vi "write read Lens Driver.vi"(0 "VISA resource name":refnum<visa-resource-name>, 5 "command":string, 7 "Calibration":T1 {"Max Current A" format="%#_g mA"; "Max Current B" format="%#_g mA"; "UCL A" format="%#_g mA"; "LCL A" format="%#_g mA"; "UCL B" format="%#_g mA"; "LCL B" format="%#_g mA"}, 11 "error in (no error)":errorcluster) -> (2 "M":i32, 4 "VISA resource name out":refnum<visa-resource-name>, 6 "Calibration 2":T1 {"Max Current A" format="%#_g mA"; "Max Current B" format="%#_g mA"; "UCL A" format="%#_g mA"; "LCL A" format="%#_g mA"; "UCL B" format="%#_g mA"; "LCL B" format="%#_g mA"}, 8 "OK":bool, 10 "Data":string, 12 "TA":u16, 13 "TB":u16, 15 "error out":errorcluster)   [LabVIEW 2024]
doc: "Basic VI to write a command to the Lens Driver and read back the answer.\nOptotune AG, 2014"
uses:
  Calibration.ctl
panel:
  out "i":i32
  out "C value":i16
  out "Number of Bytes at Serial Port":u32
  out "elapsed time (ms)":u32
  out "Response":string
  out "write":string
  out "CRC16":string
  out "read buffer":string
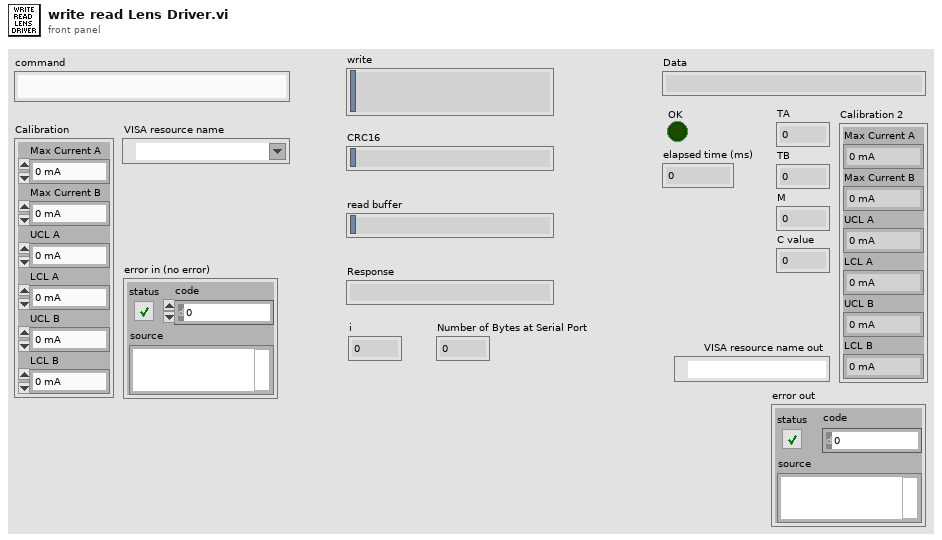
[diagram p1: front panel]
types:
  T1 = typedef "Calibration.ctl" = cluster{"Max Current A":dbl, "Max Current B":dbl, "UCL A":dbl, "UCL B":dbl, "LCL A":dbl, "LCL B":dbl}
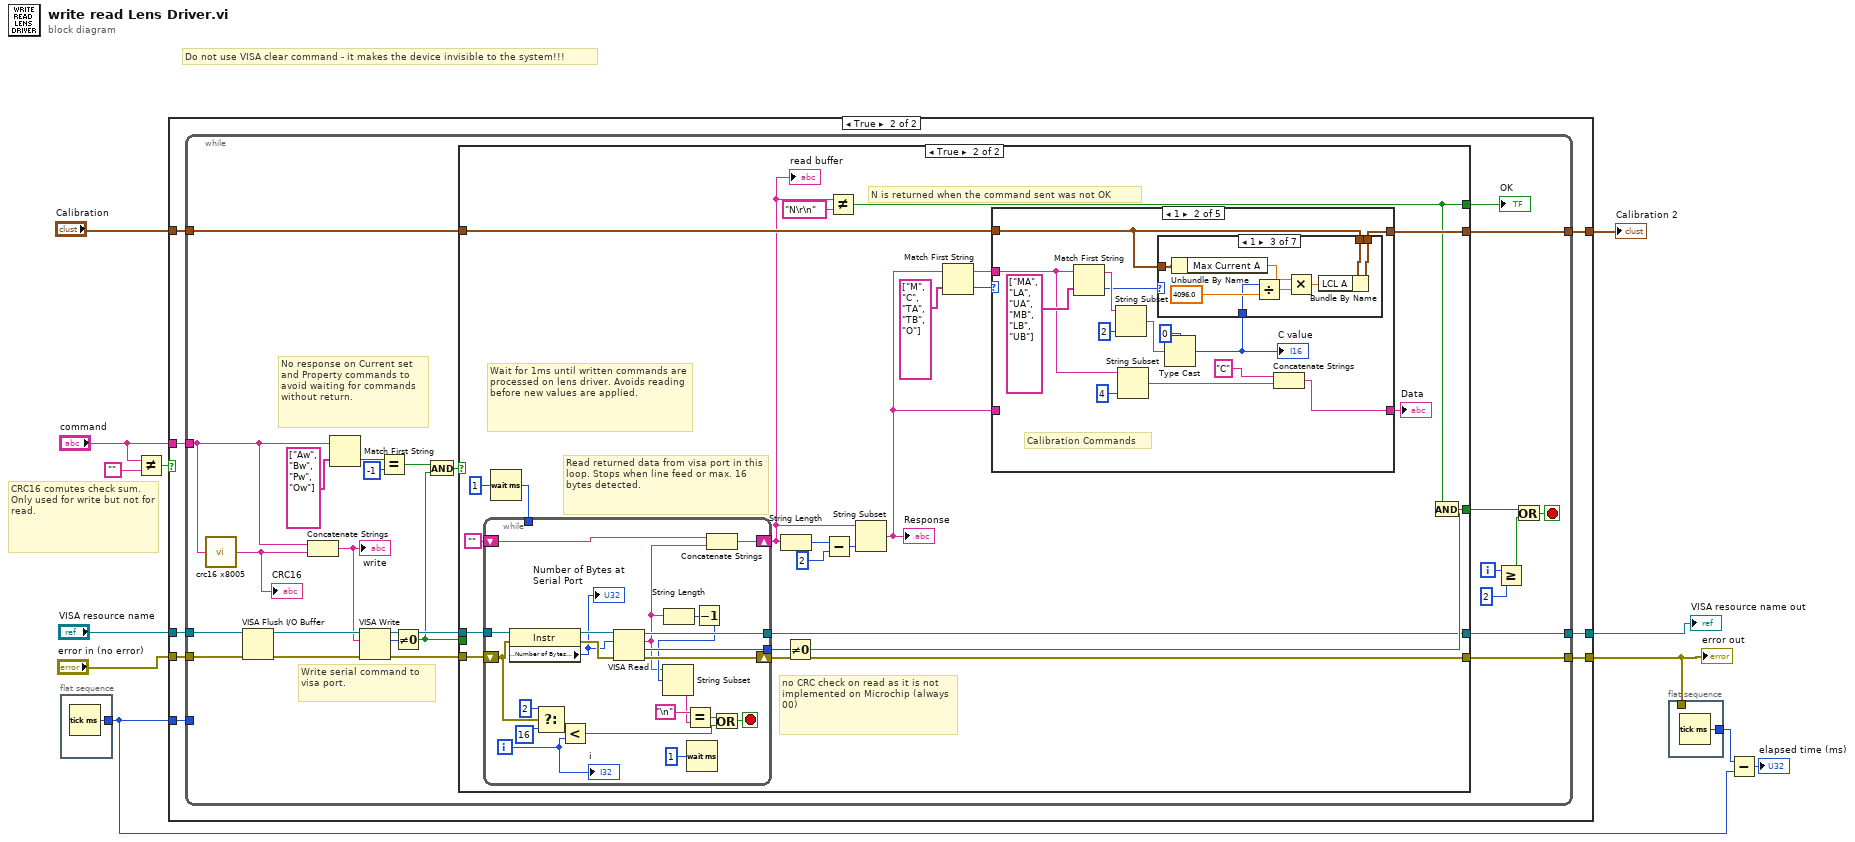
[diagram p0: block diagram]
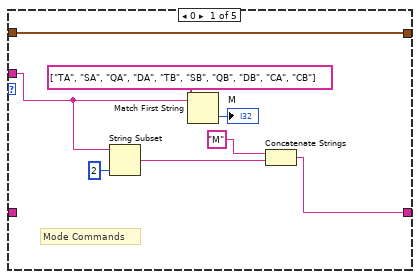
[diagram p4: hidden frame]
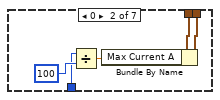
[diagram p6: hidden frame]
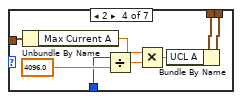
[diagram p7: hidden frame]
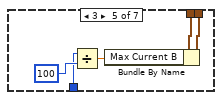
[diagram p8: hidden frame]
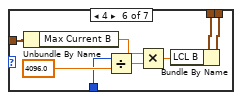
[diagram p9: hidden frame]
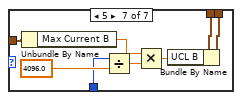
[diagram p10: hidden frame]
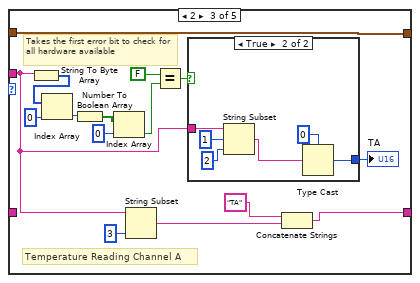
[diagram p11: hidden frame]
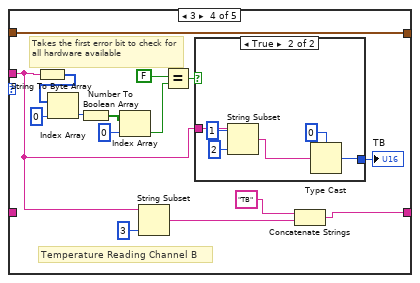
[diagram p13: hidden frame]
diagram:
  # "CRC16 comutes check sum. Only used for write but not for read."
  # "Do not use VISA clear command - it makes the device invisible to the system!!!"
  n1 = flat-sequence {
    tunnel: [w13] -> _
    tunnel: [w13] -> w10
    frame #0 {
      n2 = Tick Count (ms)() -> (millisecond timer value=w13:u32)
    }
  }
  n3 = Not Equal?(x="command", y="") -> (x != y?=w6:bool)
  n4 = case shown="True" w6 {
    tunnel: w10 -> [_ w24]
    tunnel: [w14 w23] -> w9
    tunnel: [w15 w22] -> w8
    tunnel: "Calibration" -> [w16 w21]
    tunnel: [w16 w20] -> w7
    tunnel: "command" -> [_ w19]
    tunnel: "VISA resource name" -> [w15 w18]
    tunnel: "error in (no error)" -> [w14 w17]
    frame False {
    }
    frame True {
      n5 = while {
        tunnel: w24 -> [_]
        tunnel: [w39] -> w23
        tunnel: [w35] -> w22
        tunnel: w21 -> [w30]
        tunnel: [w29] -> w20
        tunnel: w19 -> [w27]
        tunnel: w18 -> [w26]
        tunnel: w17 -> [w25]
        i -> [w33]
        stop <- w34 stop-if-true
        # "Write serial command to visa port."
        # "No response on Current set and Property commands to avoid waiting for commands without return."
        n6 = call "crc16 x8005.vi"("message"=w27) -> ("CRC16"=w45:string)  [unwired: 4 in]
        "CRC16" <- w45
        n7 = VISA Flush I/O Buffer(VISA resource name=w26, error in (no error)=w25) -> (VISA resource name out=w47:refnum<visa-resource-name>, error out=w46:errorcluster)  [unwired: 1 in]
        n8 = Concatenate Strings(w27, w45) -> (w44:string)
        "write" <- w44
        n9 = Match First String(2:string[] ["Aw", "Bw", "Pw", "Ow"] ("string array"), 3:w27) -> (0:w42:i32)  [unwired: 1 out]
        n10 = VISA Write(VISA resource name=w47, write buffer=w44, error in (no error)=w46) -> (VISA resource name out=w50:refnum<visa-resource-name>, return count=w38:u32, error out=w48:errorcluster)
        n11 = Equal?(x=w42, y=-1) -> (x = y?=w40:bool)
        n12 = Not Equal To 0?(x=w38) -> (x != 0?=w36:bool)
        n13 = And(x=w40, y=w36) -> (x .and. y?=w37:bool)
        n14 = case shown="True" w37 {
          tunnel: w50 -> [w53 w75]
          tunnel: [w51 w73] -> w49
          tunnel: w48 -> [w54 w72]
          tunnel: [w54 w69] -> w39
          tunnel: w36 -> [w51 _]
          tunnel: [w53 w63] -> w35
          tunnel: w30 -> [w52 w61]
          tunnel: [w52 w60] -> w29
          tunnel: [w51 w59] -> w28
          frame False {
          }
          frame True {
            # "Wait for 1ms until written commands are processed on lens driver. Avoids reading before new values are applied."
            # "Read returned data from visa port in this loop. Stops when line feed or max. 16 bytes detected."
            # "N is returned when the command sent was not OK"
            # "no CRC check on read as it is not implemented on Microchip (always 00)"
            n15 = Wait (ms)(milliseconds to wait=u32 1) -> (millisecond timer value=w55:u32)
            n16 = while {
              tunnel: w75 -> [w203]
              tunnel: [w208] -> w63
              shift-right: [w205] -> w57
              shift-left: "" -> [w204]
              tunnel: [w197] -> w65
              shift-right: [w209] -> w69
              shift-left: w72 -> [w193]
              tunnel: w55 -> [_]
              i -> [w199]
              stop <- w201 stop-if-true
              n17 = property class="Instr"(reference=w203, error in=w193) -> (reference out=w198:refnum<visa-resource-name>, error out=w196:errorcluster, "Serial Settings:Number of Bytes at Serial Port"=w192:u32)
              "Number of Bytes at Serial Port" <- w192
              n18 = Select(t=2, s=w193, f=16 ("x")) -> (s? t:f=w195:i32)
              n19 = Less?(x=w195, y=w199) -> (x < y?=w200:bool)
              n20 = VISA Read(VISA resource name=w198, byte count=w192, error in (no error)=w196) -> (VISA resource name out=w208:refnum<visa-resource-name>, read buffer=w188:string, return count=w197:u32, error out=w209:errorcluster)
              n21 = String Length(string=w188) -> (length=w190:i32)
              n22 = Wait (ms)(milliseconds to wait=u32 1) -> ()  [unwired: 1 out]
              n23 = Decrement(x=w190) -> (x-1=w189:i32)
              n24 = String Subset(string=w188, offset (0)=w189) -> (substring=w191:string)  [unwired: 1 in]
              n25 = Equal?(x="\n", y=w191) -> (x = y?=w206:bool)
              n26 = Concatenate Strings(w204, w188) -> (w205:string)
              n27 = Or(x=w206, y=w200) -> (x .or. y?=w201:bool)
              "i" <- w199
            }
            "read buffer" <- w57
            n28 = String Length(string=w57) -> (length=w76:i32)
            n29 = Not Equal To 0?(x=w65) -> (x != 0?=w64:bool)
            n30 = Subtract(x=w76, y=2) -> (x-y=w77:i32)
            n31 = Not Equal?(x=w57, y="N\r\n") -> (x != y?=w59:bool)
            n32 = String Subset(string=w57, length (rest)=w77) -> (substring=w58:string)  [unwired: 1 in]
            "Response" <- w58
            n33 = Match First String(2:string[] ["M", "C", "TA", "TB", "O"] ("string array"), 3:w58) -> (0:w67:i32, 1:w66:string)
            n34 = case shown="1" w67 {
              tunnel: w66 -> [w83 w93 w144 w164 _]
              tunnel: [w79 w92 w152 w173 w185] -> w62
              tunnel: [w78 w91 w151 w172 w186] -> w60
              tunnel: w61 -> [w78 w86 w151 w172 w186]
              tunnel: w58 -> [_ _ _ _ w185]
              frame 0 {
                # "Mode Commands"
                n35 = String Subset(string=w83, length (rest)=2 ("length (rest)")) -> (substring=w80:string)  [unwired: 1 in]
                n36 = Match First String(2:string[] ["TA", "SA", "QA", "DA", "TB", "SB", "QB", "DB", "CA", "CB"] ("string array"), 3:w83) -> (0:→"M":i32)  [unwired: 1 out]
                n37 = Concatenate Strings("M", w80) -> (w79:string)
              }
              frame 1 {
                # "Calibration Commands"
                n38 = Match First String(2:string[] ["MA", "LA", "UA", "MB", "LB", "UB"] ("string array"), 3:w93) -> (0:w90:i32, 1:w97:string)
                n39 = String Subset(string=w97, length (rest)=2 ("length (rest)")) -> (substring=w88:string)  [unwired: 1 in]
                n40 = String Subset(string=w93, length (rest)=4 ("length (rest)")) -> (substring=w94:string)  [unwired: 1 in]
                n41 = Type Cast(type=i16 0 ("length (rest)"), x=w88) -> (*(type *) &x=w87:i16)
                "C value" <- w87
                n42 = case shown="1" w90 {
                  tunnel: w86 -> [w100 w105 w113 w121 w126 w134 w142]
                  tunnel: [w100 w104 w112 w120 w125 w133 w141] -> w91
                  tunnel: w87 -> [_ w102 w106 w114 w122 w127 w135]
                  tunnel: w86 -> [_ _ w111 w115 _ w128 w136]
                  frame -1, Default {
                  }
                  frame 0 {
                    n43 = Divide(x=w102, y=u16 100) -> (x/y=w101:dbl)
                    n44 = Bundle By Name(cluster=w105, "Max Current A"=w101) -> (w104:T1)
                  }
                  frame 1 {
                    n45 = Unbundle By Name(w111) -> ("Max Current A"=w109:dbl)
                    n46 = Divide(x=w106, y=4096.0) -> (x/y=w107:dbl)
                    n47 = Multiply(x=w109, y=w107) -> (x*y=w108:dbl)
                    n48 = Bundle By Name(cluster=w113, "LCL A"=w108) -> (w112:T1)
                  }
                  frame 2 {
                    n49 = Unbundle By Name(w115) -> ("Max Current A"=w118:dbl)
                    n50 = Divide(x=w114, y=4096.0) -> (x/y=w117:dbl)
                    n51 = Multiply(x=w118, y=w117) -> (x*y=w116:dbl)
                    n52 = Bundle By Name(cluster=w121, "UCL A"=w116) -> (w120:T1)
                  }
                  frame 3 {
                    n53 = Divide(x=w122, y=u16 100) -> (x/y=w124:dbl)
                    n54 = Bundle By Name(cluster=w126, "Max Current B"=w124) -> (w125:T1)
                  }
                  frame 4 {
                    n55 = Unbundle By Name(w128) -> ("Max Current B"=w131:dbl)
                    n56 = Divide(x=w127, y=4096.0) -> (x/y=w130:dbl)
                    n57 = Multiply(x=w131, y=w130) -> (x*y=w129:dbl)
                    n58 = Bundle By Name(cluster=w134, "LCL B"=w129) -> (w133:T1)
                  }
                  frame 5 {
                    n59 = Unbundle By Name(w136) -> ("Max Current B"=w139:dbl)
                    n60 = Divide(x=w135, y=4096.0) -> (x/y=w140:dbl)
                    n61 = Multiply(x=w139, y=w140) -> (x*y=w137:dbl)
                    n62 = Bundle By Name(cluster=w142, "UCL B"=w137) -> (w141:T1)
                  }
                }
                n63 = Concatenate Strings("C", w94) -> (w92:string)
              }
              frame 2 {
                # "Takes the first error bit to check for all hardware available"
                # "Temperature Reading Channel A"
                n64 = String To Byte Array(string=w144) -> (unsigned byte array=w149:u8[])
                n65 = Index Array(array=w149, index=0) -> (element=w148:u8)
                n66 = Number To Boolean Array(number=w148) -> (Boolean array=w146:bool[])
                n67 = Index Array(array=w146, index=0) -> (element=w143:bool)
                n68 = String Subset(string=w144, length (rest)=3 ("length (rest)")) -> (substring=w153:string)  [unwired: 1 in]
                n69 = Equal?(x=FALSE, y=w143) -> (x = y?=w157:bool)
                n70 = case shown="True" w157 {
                  tunnel: w144 -> [_ w162]
                  tunnel: [_ w159] -> w156
                  frame False {
                  }
                  frame True {
                    n71 = String Subset(string=w162, offset (0)=1, length (rest)=2 ("length (rest)")) -> (substring=w158:string)
                    n72 = Type Cast(type=u16 0 ("length (rest)"), x=w158) -> (*(type *) &x=w159:u16)
                  }
                }
                "TA" <- w156
                n73 = Concatenate Strings("TA", w153) -> (w152:string)
              }
              frame 3 {
                # "Takes the first error bit to check for all hardware available"
                # "Temperature Reading Channel B"
                n74 = String To Byte Array(string=w164) -> (unsigned byte array=w170:u8[])
                n75 = Index Array(array=w170, index=0) -> (element=w169:u8)
                n76 = Number To Boolean Array(number=w169) -> (Boolean array=w168:bool[])
                n77 = Index Array(array=w168, index=0) -> (element=w165:bool)
                n78 = String Subset(string=w164, length (rest)=3 ("length (rest)")) -> (substring=w174:string)  [unwired: 1 in]
                n79 = Equal?(x=FALSE, y=w165) -> (x = y?=w178:bool)
                n80 = case shown="True" w178 {
                  tunnel: w164 -> [_ w183]
                  tunnel: [_ w180] -> w177
                  frame False {
                  }
                  frame True {
                    n81 = String Subset(string=w183, offset (0)=1, length (rest)=2 ("length (rest)")) -> (substring=w179:string)
                    n82 = Type Cast(type=u16 0 ("length (rest)"), x=w179) -> (*(type *) &x=w180:u16)
                  }
                }
                "TB" <- w177
                n83 = Concatenate Strings("TB", w174) -> (w173:string)
              }
              frame -1, Default {
              }
            }
            "Data" <- w62
            n84 = And(x=w59, y=w64) -> (x .and. y?=w73:bool)
          }
        }
        "OK" <- w28
        n85 = Greater Or Equal?(x=w33, y=2) -> (x >= y?=w31:bool)
        n86 = Or(x=w49, y=w31) -> (x .or. y?=w34:bool)
      }
    }
  }
  "error out" <- w9
  "VISA resource name out" <- w8
  "Calibration 2" <- w7
  n87 = flat-sequence {
    tunnel: [w210] -> w11
    tunnel: w9 -> [_]
    frame #0 {
      n88 = Tick Count (ms)() -> (millisecond timer value=w210:u32)
    }
  }
  n89 = Subtract(x=w11, y=w10) -> (x-y=→"elapsed time (ms)":u32)
